vi "SOUR_POW_CORR_COLL_BSEN_FRAN.vi"(0 "VISA IN":refnum<visa-resource-name>, 5 "error in":errorcluster, 7 "Channel":i32) -> (14 "VISA Out":refnum<visa-resource-name>, 16 "Data":string, 19 "error out":errorcluster)   [LabVIEW 2018, in "PNA-X.lvlib"]
doc: "SOURce:POWer:CORRection:COLLect:BSENsor[:FRANge]? \nReturn Type Numeric \nDefault 0,0 \nSOURce<cnum>:POWer:CORRection:COLLect:<pmChan>SENsor:RCFactor <num> \n(Read-Write) ) Specifies the reference cal factor for the power sensor connected to channel A or B of \nthe power meter. If the power meter has only a single channel, that channel is considered channel A. \nNote: If the sensor connected to the specified channel of the power meter contains cal factors in \nEPROM (such as the Agilent E-series power sensors), those will be the cal factors used during the \ncalibration sweep. The reference cal factor value associated with this command, and any cal factors \nentered into the PNA for that sensor channel, will not be used. \nParameters \n<cnum> Any existing channel number. If unspecified, value is set to 1 \n<pmChan> Power Meter channel. Choose from: \nA - Channel A \nB - Channel B \n1842\n\n<num> Reference cal factor in percent. Choose any number between 1 and 150. \nExamples SOUR:POW:CORR:COLL:ASEN:RCF 98.7 \nsource1:power2:correction:collect:bsensor:rcfactor 105 \nQuery Syntax SOURce:POWer:CORRection:COLLect:ASENsor:RCFactor?"
uses:
  PNA-X.lvlib
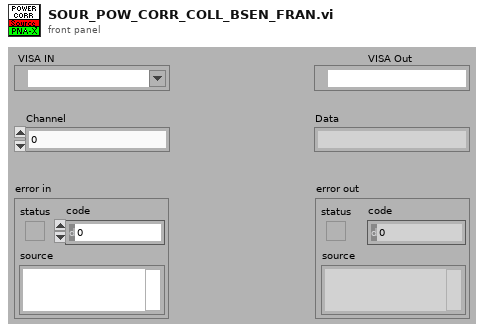
[diagram p1: front panel]
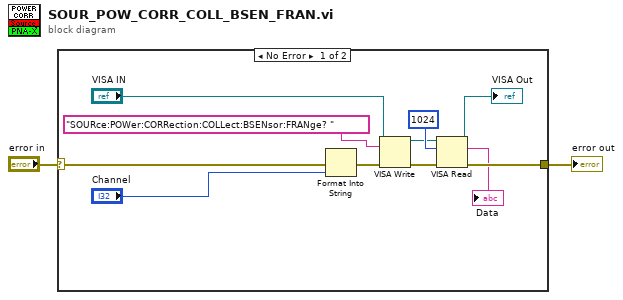
[diagram p0: block diagram]
diagram:
  n1 = case shown="No Error" "error in" {
    selector: "error in" -> [w13 w14]
    tunnel: [w7 w14] -> w1
    frame No Error {
      n2 = Format Into String(error in=w13, "Channel") -> (error out=w12:errorcluster)  [unwired: 2 in, 1 out]
      n3 = VISA Write(VISA resource name="VISA IN", write buffer="SOURce:POWer:CORRection:COLLect:BSENsor:FRANge? " ("Cmdline"), error in (no error)=w12) -> (VISA resource name out=w8:refnum<visa-resource-name>, error out=w10:errorcluster)  [unwired: 1 out]
      n4 = VISA Read(VISA resource name=w8, byte count=1024, error in (no error)=w10) -> (VISA resource name out=→"VISA Out":refnum<visa-resource-name>, read buffer=→"Data":string, error out=w7:errorcluster)  [unwired: 1 out]
    }
    frame Error {
    }
  }
  "error out" <- w1
